vi "_FPGA_StepwiseScan_DataReader.vi"(8 "Read data":bool, 11 "Data in":u64) -> (0 "End?":bool, 1 "Valid?":bool, 2 "Timed Out?":bool, 3 "Data out":u64)   [LabVIEW 2018]
uses:
  <vilib>/rvi/DataTransferAndStorage/Container/XNode/niFpgaContainer.xnode
  <vilib>/rvi/interface/RandomDataEmulation/nirviRandomDataFpgaReadWriteTemplate.vi
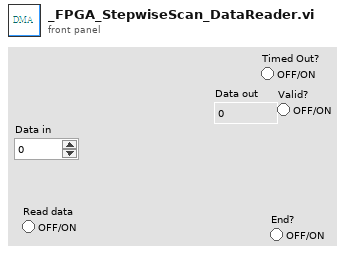
[diagram p1: front panel]
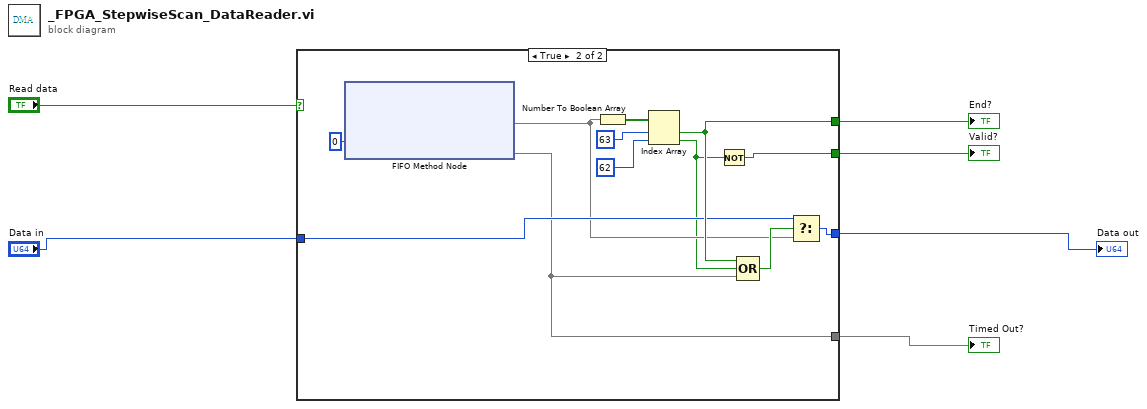
[diagram p0: block diagram]
diagram:
  n1 = case shown="True" "Read data" {
    tunnel: [_ w8] -> w1
    tunnel: [w7 w14] -> w3
    tunnel: "Data in" -> [w7 w12]
    tunnel: [_ w15] -> w5
    tunnel: [_ w10] -> w4
    frame False {
    }
    frame True {
      n2 = xnode ("FIFO Method Node")("Timeout"=0) -> ("Element"=w11, "Timed Out?"=w8)  [unwired: 1 in, 1 out]
      n3 = Number To Boolean Array(number=w11) -> (Boolean array=w17:bool[])
      n4 = Index Array(array=w17, index #1=63 ("index"), index #2=62 ("index")) -> (element #1=w15:bool, element #2=w9:bool)
      n5 = Not(x=w9) -> (.not. x?=w10:bool)
      n6 = Compound Arithmetic op=OR(w15, w9, w8) -> (w13:bool)
      n7 = Select(t=w12, s=w13, f=w11) -> (s? t:f=w14:u64)
    }
  }
  "End?" <- w5
  "Timed Out?" <- w1
  "Data out" <- w3
  "Valid?" <- w4
